vi "阀口名称设置.vi"() -> ()   [LabVIEW 2016, in "斯坦道总氮.lvlib"]
panel:
  in  "取消":bool
  in  "确认":bool
  in  "阀口名称":T1={"V"="试剂1", "V 2"="试剂2", "V 3"="试剂3", "V 4"="试剂4", "V 5"="试剂5", "V 6"="试剂6", "V 7"="试剂7", "V 8"="试剂8", "V 9"="试剂9", "V 10"="试剂10", "V 11"="试剂11", "V 12"="试剂12", "V9-1"="试剂13", "V9-2"="试剂14"}
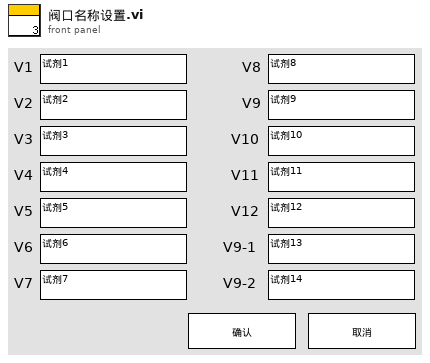
[diagram p1: front panel]
types:
  T1 = cluster{"V":string, "V 2":string, "V 3":string, "V 4":string, "V 5":string, "V 6":string, "V 7":string, "V 8":string, "V 9":string, "V 10":string, "V 11":string, "V 12":string, "V9-1":string, "V9-2":string}
  T2 = cluster{"时间标识":timestamp, "设备":string, "日志信息":string, "流程参数":string}
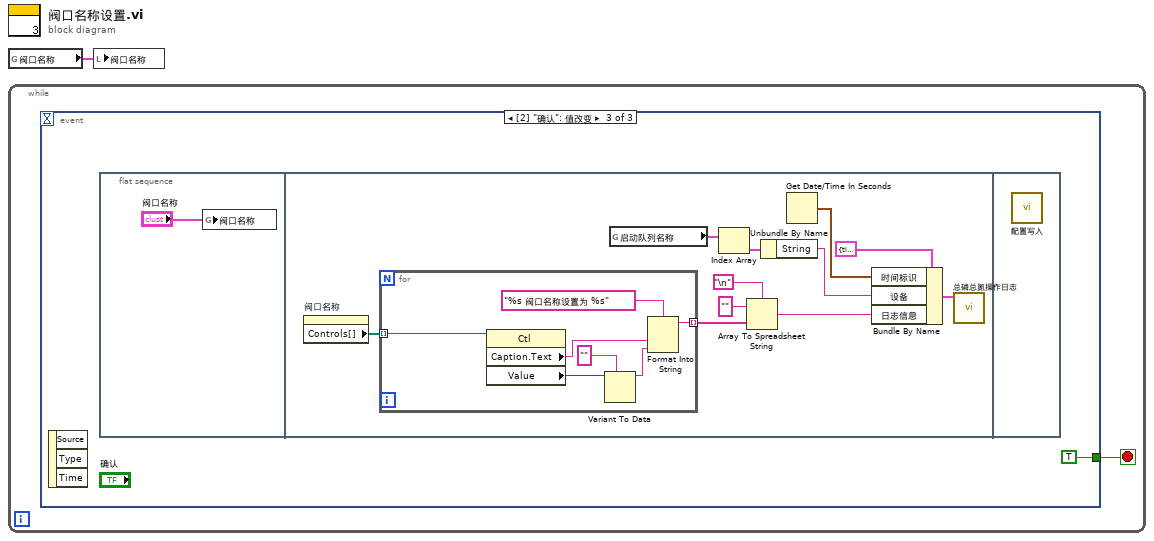
[diagram p0: block diagram]
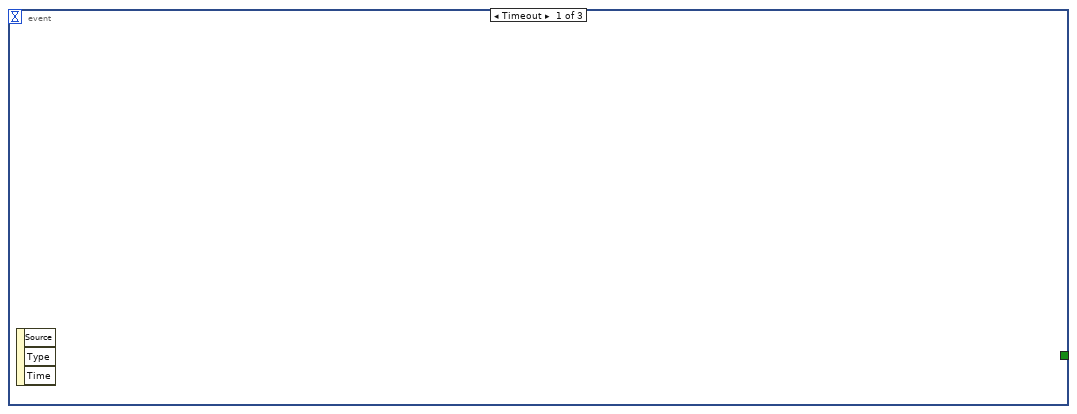
[diagram p2: hidden frame]
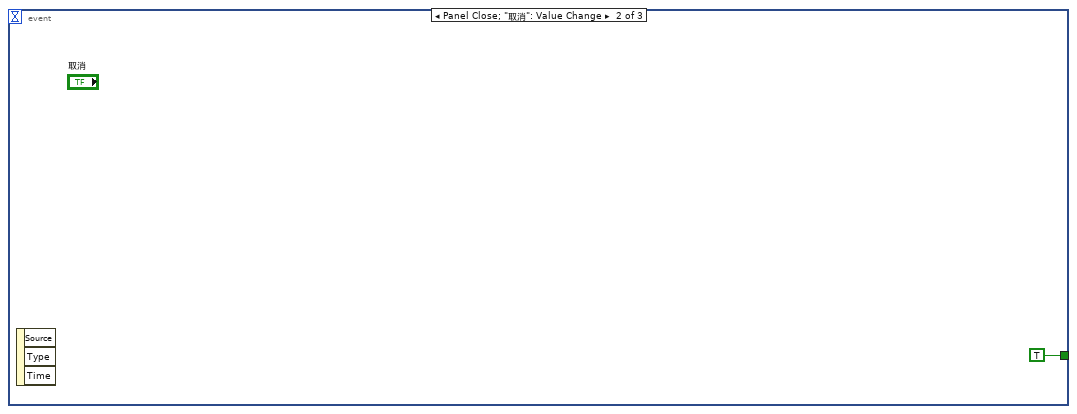
[diagram p3: hidden frame]
diagram:
  n1 = global read "总磷总氮断电保存全局变量.vi" "阀口名称"() -> (w1:T1)
  n2 = while {
    stop <- w2 stop-if-true
    n3 = event shown="[2] \"确认\": 值改变" {
      selector: _ -> [_ _ _]
      dyn-events: _ -> [_ _ _]
      timeout: _ -> [_ _ _]
      tunnel: [_ TRUE TRUE] -> w2
      event Timeout {
        n4 = event-data() -> ()  [unwired: 1 in, 3 out]
      }
      event Panel Close; "取消": Value Change {
        n5 = event-data() -> ()  [unwired: 1 in, 3 out]
      }
      event "确认": Value Change {
        n6 = event-data() -> ()  [unwired: 1 in, 3 out]
        n7 = flat-sequence {
          frame #0 {
            n8 = global write "总磷总氮断电保存全局变量.vi" "阀口名称"("阀口名称") -> ()
          }
          frame #1 {
            n9 = property on="阀口名称" class="Clust (严格)"() -> ("Controls[]"=w10:refnum<vi>[])  [unwired: 2 in, 2 out]
            n10 = for {
              tunnel: w10 -> [w23] mode=indexing
              tunnel: [w18] -> w9 mode=indexing
              n11 = property class="Ctl"(reference=w23) -> ("Caption.Text"=w22:string, "Value"=w20:variant)  [unwired: 1 in, 2 out]
              n12 = Variant To Data(type="", Variant=w20) -> (data=w19:string)  [unwired: 1 in, 1 out]
              n13 = Format Into String(format string="%s 阀口名称设置为 %s" ("格式字符串"), w22, w19) -> (resulting string=w18:string)  [unwired: 2 in, 1 out]
            }
            n14 = global read "总磷总氮断电保存全局变量.vi" "启动队列名称"() -> (w14:cluster{"String":string, "Value":u16}[])
            n15 = Index Array(array=w14) -> (element=w15:cluster{"String":string, "Value":u16})  [unwired: 1 in]
            n16 = Array To Spreadsheet String(delimiter (Tab)="\n", array=w9, 3:"" ("格式字符串")) -> (spreadsheet string=w7:string)
            n17 = Unbundle By Name(w15) -> ("String"=w16:string)
            n18 = Get Date/Time In Seconds() -> (seconds since 1Jan1904=w13:timestamp)
            n19 = Bundle By Name(cluster=T2 {"时间标识"=timestamp(0 s since 1904-01-01), "设备"="", "日志信息"="", "流程参数"=""} ("data in"), "时间标识"=w13, "设备"=w16, "日志信息"=w7) -> (w12:T2)
            n20 = call "总磷总氮操作日志.vi"("data in"=w12) -> ()  [unwired: 11 in]
          }
          frame #2 {
            n21 = call "配置写入.vi"() -> ()  [unwired: 11 in, 1 out]
          }
        }
      }
    }
  }
  n22 = local write "阀口名称"(w1) -> ()
